vi "from string.vi"(8 "error in":errorcluster, 9 "channel data":string, 10 "identifier":string, 11 "channel in":refnum<class "EIP Tags Channel.lvclass">) -> (0 "error out":errorcluster, 3 "channel out":refnum<class "EIP Tags Channel.lvclass">)   [LabVIEW 2013, in "EIP Tags Channel.lvclass"]
doc: "NI Tag Bus Module Framework 1.0.3.46\nNI Systems Engineering"
uses:
  EIP Tags Channel.lvclass
  <vilib>/NI/Tag Bus/tag/Data Type.ctl
  <vilib>/NI/Tag Bus Module Framework/channel/channel classification.ctl
  <vilib>/NI/Tag Bus/tag/tag descriptor.lvclass/tag descriptor.ctl
  <vilib>/NI/Tag Bus Module Framework/channel/TBM channel.lvclass/TBM channel.ctl
  EIP Tags Channel.lvclass/EIP Tags Channel.ctl
  <vilib>/NI/Tag Bus/tag/tag descriptor.lvclass
  <vilib>/NI/Tag Bus Module Framework/channel/TBM channel.lvclass
  <vilib>/NI/Configuration Framework/serializable configuration/NISE_CEF_serializable configuration.lvclass
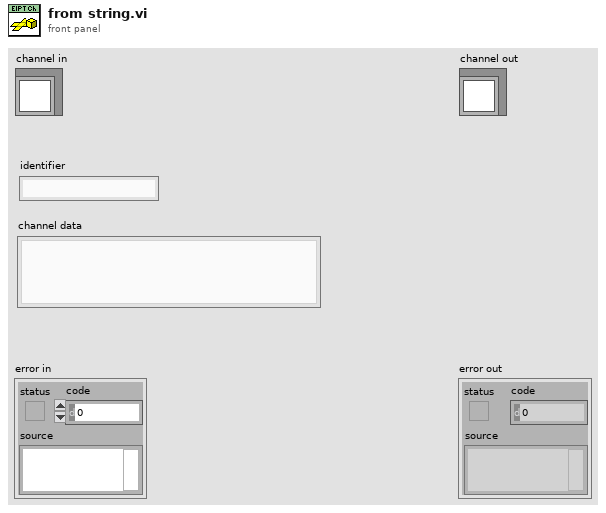
[diagram p1: front panel]
types:
  T1 = typedef "TBM channel.lvclass/channel classification.ctl" = enum16{"input data", "output data", "processing parameter", "processing result"}
  T2 = typedef "tag bus.lvlib/tag descriptor.lvclass/Data Type.ctl" = enum16{"Double", "Single", "I64", "I32", "I16", "I8", "U64", "U32", "U16", "U8", "Boolean", "String", "Array of Double", "Array of Single", "Array of I64", "Array of I32", "Array of I16", "Array of I8", "Array of U64", "Array of U32", "Array of U16", "Array of U8", "Array of Boolean", "Array of String"}
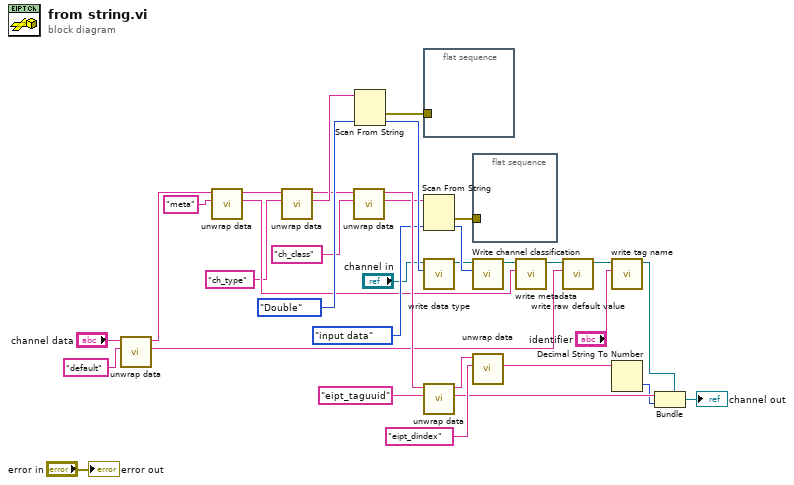
[diagram p0: block diagram]
diagram:
  n1 = call <vilib>:"unwrap data.vi"("identifier"="default", "data to unwrap"="channel data") -> ("unwrapped data"=w15:string, "remaining string"=w6:string)  [unwired: 8 in]
  n2 = call <vilib>:"unwrap data.vi"("identifier"="meta", "data to unwrap"=w6) -> ("unwrapped data"=w14:string, "remaining string"=w10:string)  [unwired: 8 in]
  n3 = call <vilib>:"unwrap data.vi"("identifier"="ch_type", "data to unwrap"=w10) -> ("unwrapped data"=w16:string, "remaining string"=w9:string)  [unwired: 8 in]
  n4 = call <vilib>:"unwrap data.vi"("identifier"="ch_class", "data to unwrap"=w9) -> ("unwrapped data"=w18:string, "remaining string"=w28:string)  [unwired: 8 in]
  n5 = Scan From String(input string=w16, default 1=Data_Type."Double" ("data type")) -> (error out=w20:errorcluster, output 1=w24:T2)  [unwired: 3 in, 2 out]
  n6 = flat-sequence {
    tunnel: w20 -> [_]
    frame #0 {
    }
  }
  n7 = Scan From String(input string=w18, default 1=channel_classification."input data" ("channel classification")) -> (error out=w21:errorcluster, output 1=w26:T1)  [unwired: 3 in, 2 out]
  n8 = call <vilib>:"write data type.vi"("data type"=w24, "system tag in"="channel in") -> ("system tag out"=w23:refnum<class "EIP Tags Channel.lvclass">)  [unwired: 8 in, 1 out]
  n9 = call <vilib>:"unwrap data.vi"("identifier"="eipt_taguuid", "data to unwrap"=w28) -> ("unwrapped data"=w3:string, "remaining string"=w2:string)  [unwired: 8 in]
  n10 = flat-sequence {
    tunnel: w21 -> [_]
    frame #0 {
    }
  }
  n11 = call <vilib>:"Write channel classification.vi"("channel classification"=w26, "channel in"=w23) -> ("channel out"=w25:refnum<class "EIP Tags Channel.lvclass">)  [unwired: 8 in, 1 out]
  n12 = call <vilib>:"unwrap data.vi"("identifier"="eipt_dindex", "data to unwrap"=w2) -> ("unwrapped data"=w30:string)  [unwired: 8 in, 1 out]
  n13 = call <vilib>:"write metadata.vi"("metadata"=w14, "system tag in"=w25) -> ("system tag out"=w13:refnum<class "EIP Tags Channel.lvclass">)  [unwired: 8 in, 1 out]
  n14 = call <vilib>:"write raw default value.vi"("raw default"=w15, "system tag in"=w13) -> ("system tag out"=w22:refnum<class "EIP Tags Channel.lvclass">)  [unwired: 8 in, 1 out]
  n15 = call <vilib>:"write tag name.vi"("name"="identifier", "system tag in"=w22) -> ("system tag out"=w31:refnum<class "EIP Tags Channel.lvclass">)  [unwired: 8 in, 1 out]
  n16 = Decimal String To Number(string=w30) -> (number=w1:i32)  [unwired: 2 in, 1 out]
  n17 = Bundle(cluster=w31, w3, w1) -> (→"channel out":refnum<class "EIP Tags Channel.lvclass">)
  "error out" <- "error in"
